vi "HEWH Solenoid Output Set.vi"(8 "Error In":errorcluster, 9 "HEWH MW100 Channel Numbers":T2="011", 10 "Outlet Valve":T1="OFF", 11 "VISA session":refnum<visa-resource-name>="MW100") -> (0 "Error Out":errorcluster, 3 "dup VISA session":refnum<visa-resource-name>)   [LabVIEW 2016]
uses:
  Type Definitions/HEWH MW100 Channel Numbers.ctl
  Type Definitions/HEWH Normally Open Valve Control.ctl
panel:
  out "Message":string
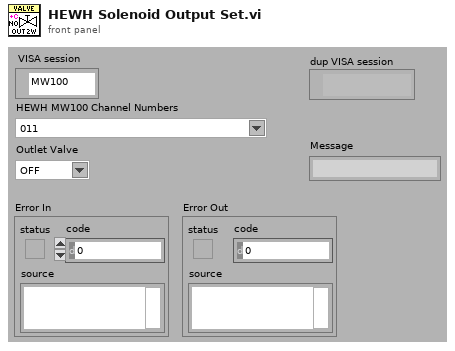
[diagram p1: front panel]
types:
  T1 = typedef "HEWH Normally Open Valve Control.ctl" = string
  T2 = typedef "HEWH MW100 Channel Numbers.ctl" = string
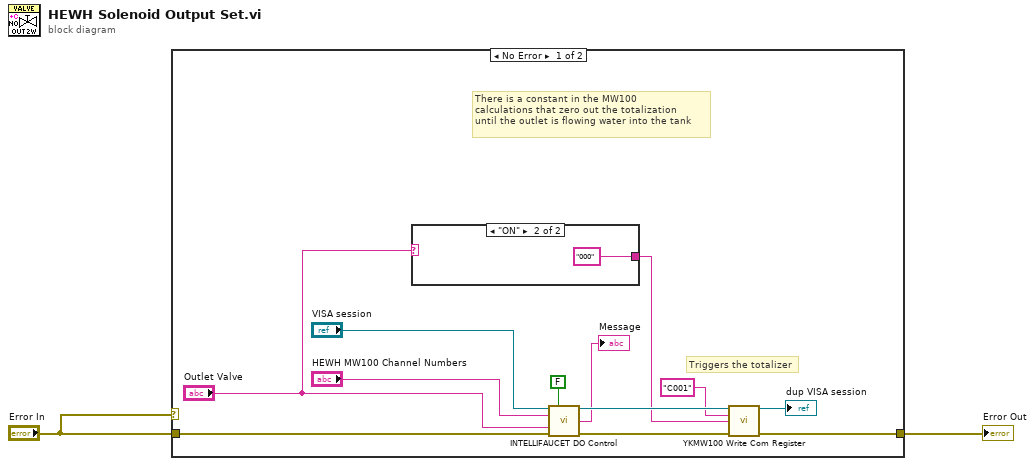
[diagram p0: block diagram]
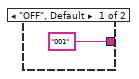
[diagram p2: hidden frame]
diagram:
  n1 = case shown="No Error" "Error In" {
    selector: "Error In" -> [_ w17]
    tunnel: "Error In" -> [w8 _]
    tunnel: [w7 w17] -> w2
    frame No Error {
      # "There is a constant in the MW100\ncalculations that zero out the totalization\nuntil the outlet is flowing water into the tank"
      # "Triggers the totalizer"
      n2 = case shown="\"ON\"" "Outlet Valve" {
        tunnel: ["001" ("Channel") "000" ("Channel")] -> w9
        frame "OFF", Default {
        }
        frame "ON" {
        }
      }
      n3 = call "INTELLIFAUCET DO Control.vi"("VISA session"="VISA session", "Normally Closed Valve?"=FALSE, "HEWH MW100 Channel Numbers"="HEWH MW100 Channel Numbers", "Normally Open Valve"="Outlet Valve", "Error In"=w8) -> ("dup VISA session"=w11:refnum<visa-resource-name>, "Message"=→"Message":string, "error out"=w13:errorcluster)  [unwired: 7 in, 1 out]
      n4 = call "YKMW100 Write Com Register.vi"("VISA session"=w11, "Channel"="C001", "Value"=w9, "error in (no error)"=w13) -> ("dup VISA session"=→"dup VISA session":refnum<visa-resource-name>, "error out"=w7:errorcluster)  [unwired: 10 in]
    }
    frame Error {
    }
  }
  "Error Out" <- w2
